vi "Hi_Tec_Control.vi"(2 "Carrier 1_50 Voltage":dbl(knob) min=0.0 max=5.0 scale=0.0..5.0 scale format="%.1f", 3 "Client Name":string, 4 "Trace_2 Voltage":dbl(knob) min=0.0 max=5.0 scale=0.0..5.0 scale format="%.1f", 5 "Trace Voltage":dbl(knob) min=0.0 max=5.0 scale=0.0..5.0 scale format="%.1f", 6 "Carrier 2 Voltage":dbl(knob) min=0.0 max=5.0 scale=0.0..5.0 scale format="%.1f", 7 "Carrier 1 Voltage":dbl(knob) min=0.0 max=5.0 scale=0.0..5.0 scale format="%.1f") -> (1 "Scan Comments":string)   [LabVIEW 2018]
uses:
  ADAM Client/Sub VIs/Channel_State_Control.ctl
  Anemometry/Anemometry Sub Vis/Controls/In_Range.ctl
  ADAM Client/Sub VIs/ADAM Controls/Update_scan_value.ctl
panel:
  out "Second stage":dbl[][](graph)
  out "First stage":dbl[][](graph)
  out "Increasing trace":bool
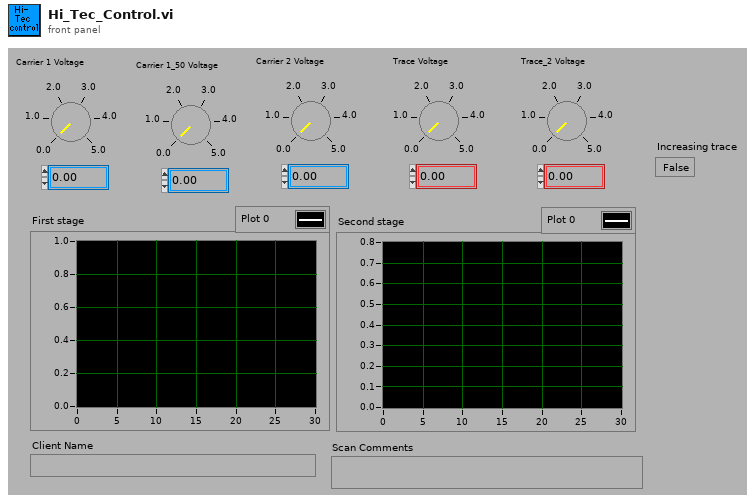
[diagram p1: front panel]
types:
  T1 = typedef "Channel_State_Control.ctl" = enum16{"Channel Name", "Channel Name Starts with", "Main Address"}
  T2 = typedef "In_Range.ctl" = enum16{"%", "±", "% & ±"}
  T3 = typedef "Update_scan_value.ctl" = cluster{"Channel Name":string, "New Value":dbl}
  T4 = enum16{"Append to Global", "Read Global then Clear"}
  T5 = typedef "Ch_description_ADAM.ctl" = cluster{"Ch Name":string, "Type":T6, "Function":T7, "Ch State":T8, "Calibration type":T9, "A":dbl, "B":dbl, "C":dbl, "D":dbl, "Comments":string, "Address":T10, "String":string, "Duty":u16}
  T6 = typedef "Module_type_ADAM.ctl" = string
  T7 = typedef "Function_ADAM.ctl" = enum16{"Analogue Input", "Digital Input", "Event counter", "Event rate", "Analogue Output", "Digital Output", "Relay Output"}
  T8 = typedef "Channel_State.ctl" = enum16{"On", "Off", "Always On", "Always Off"}
  T9 = typedef "Calib_type_ADAM.ctl" = string
  T10 = typedef "Address.ctl" = cluster{"Main":i32, "Ch.":i32, "Sub":i32, "Port Name":string}
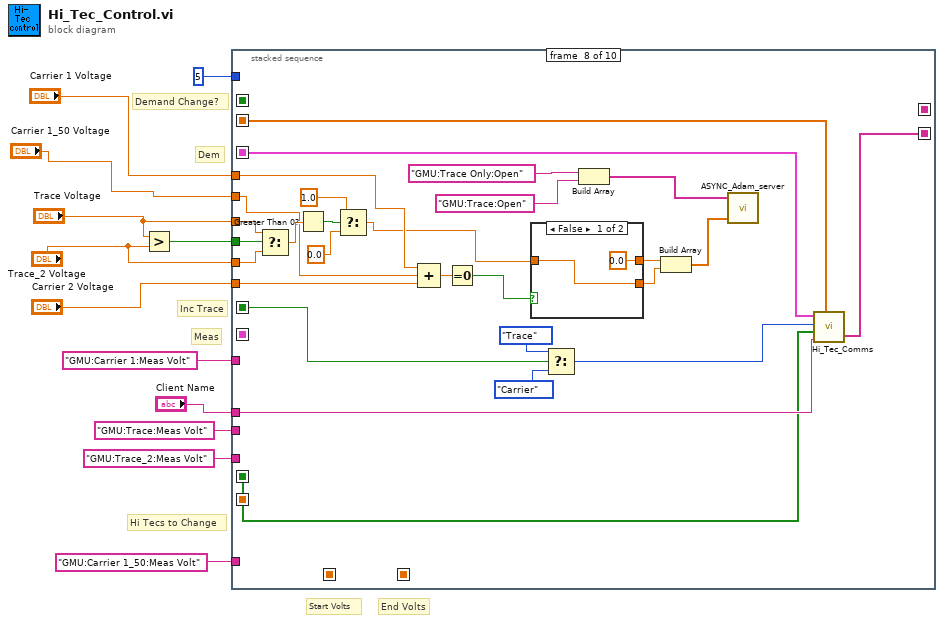
[diagram p0: block diagram]
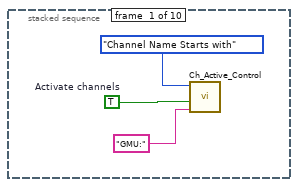
[diagram p2: hidden frame]
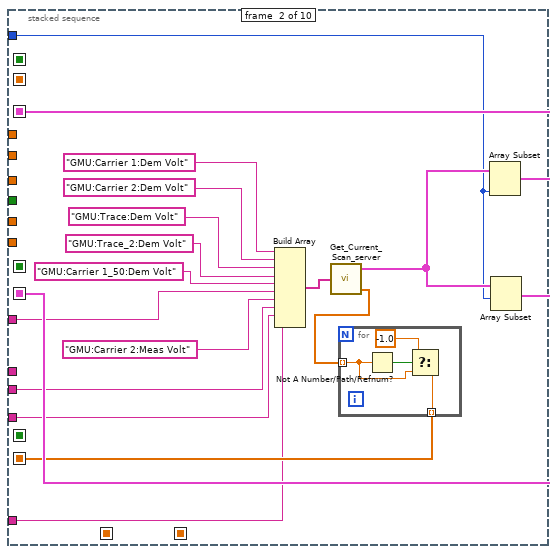
[diagram p3: hidden frame]
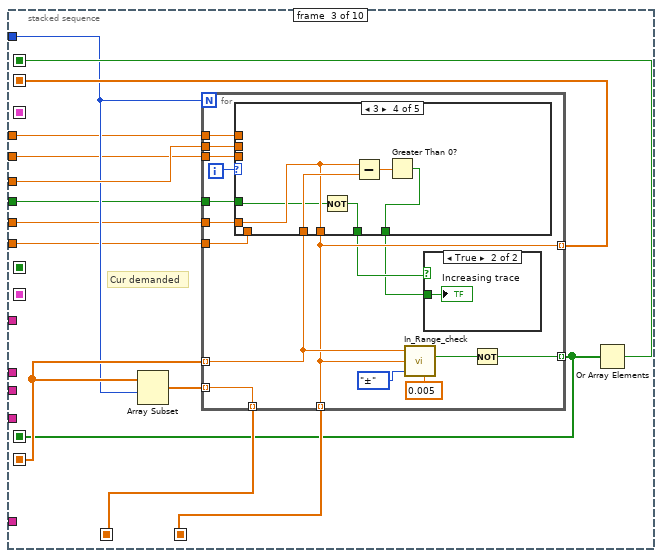
[diagram p4: hidden frame]
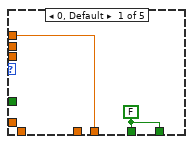
[diagram p6: hidden frame]
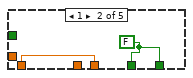
[diagram p7: hidden frame]
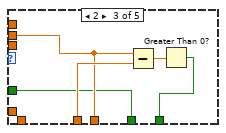
[diagram p8: hidden frame]
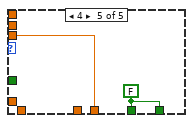
[diagram p9: hidden frame]
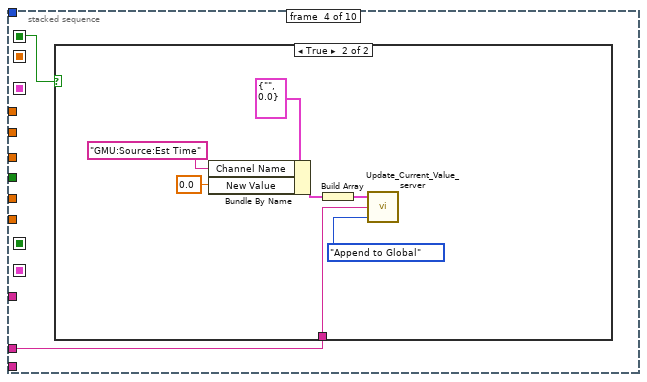
[diagram p10: hidden frame]
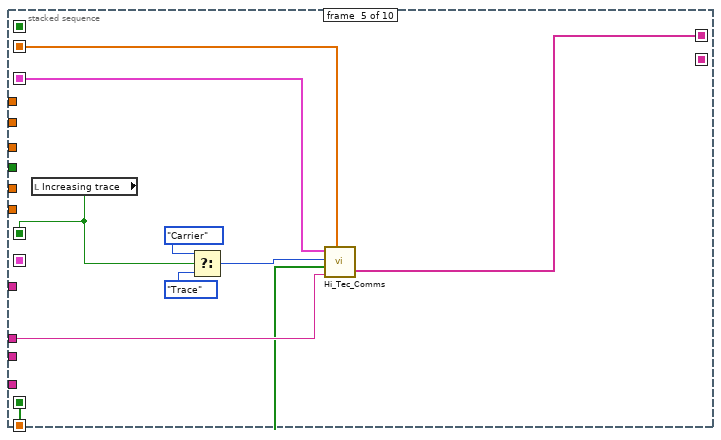
[diagram p12: hidden frame]
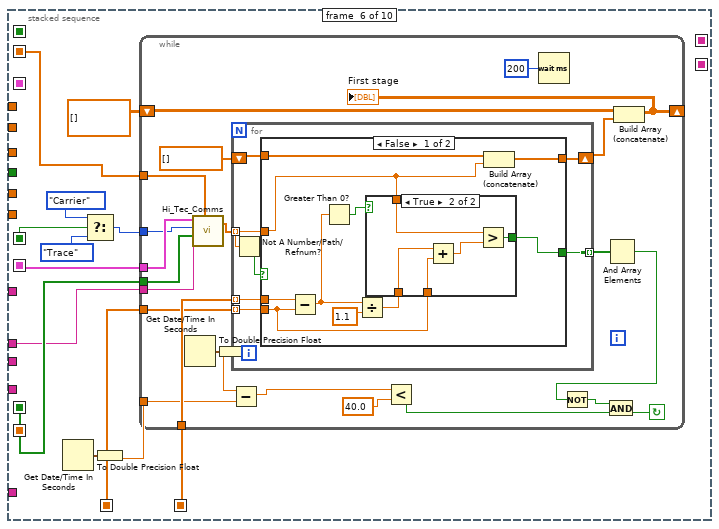
[diagram p13: hidden frame]
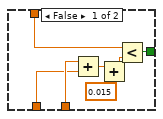
[diagram p14: hidden frame]
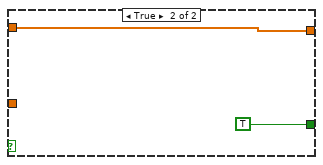
[diagram p15: hidden frame]
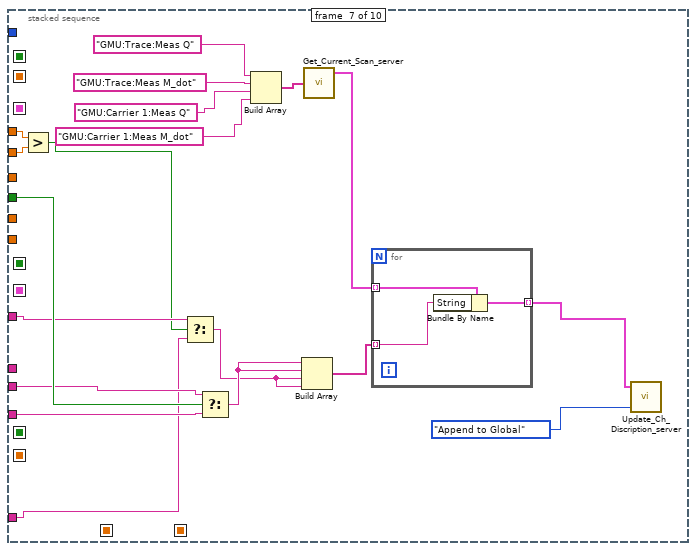
[diagram p16: hidden frame]
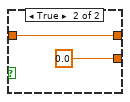
[diagram p17: hidden frame]
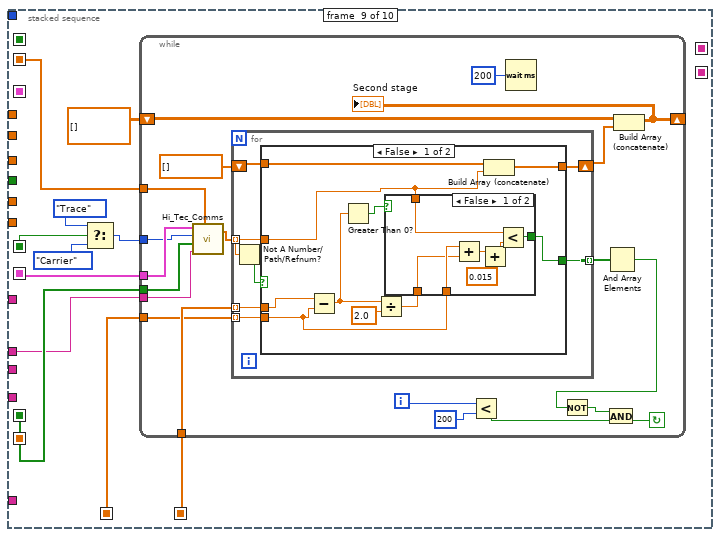
[diagram p18: hidden frame]
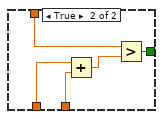
[diagram p19: hidden frame]
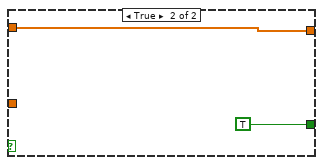
[diagram p20: hidden frame]
diagram:
  # "Dem"
  # "Demand Change?"
  # "End Volts"
  # "Start Volts"
  # "Inc Trace"
  # "Meas"
  # "Hi Tecs to Change"
  n1 = Greater?(x="Trace Voltage", y="Trace_2 Voltage") -> (0:w9:bool)
  n2 = stacked-sequence {
    seq-local: [_ w28 _ _ _ _ _ _ _ _] -> [_ _ _ _ w96 _ _ w208 _ w289]
    seq-local: [_ w23 _ _ _ _ _ _ _ _] -> [_ _ w48 _ _ _ _ _ _ _]
    seq-local: [_ _ w46 _ _ _ _ _ _ _] -> [_ _ _ _ w95 w115 _ w207 w234 _]
    seq-local: [_ w27 _ _ _ _ _ _ _ _] -> [_ _ _ _ _ w111 _ _ w230 _]
    seq-local: [_ _ _ _ w102 _ _ _ _ _] -> [_ _ _ _ _ w112 _ w219 w231 _]
    seq-local: [_ _ w50 _ _ _ _ _ _ _] -> [_ _ _ _ _ w108 _ _ w227 _]
    seq-local: [_ _ w49 _ _ _ _ _ _ _] -> [_ _ _ _ _ w109 _ _ w228 _]
    seq-local: [_ _ w45 _ _ _ _ _ _ _] -> [_ _ _ w85 _ _ _ _ _ _]
    seq-local: [_ _ w43 _ _ _ _ _ _ _] -> [_ _ _ _ w97 w103 _ w209 w224 w288]
    seq-local: [_ _ _ _ w94 _ _ _ _ _] -> [_ _ _ _ _ _ _ _ _ _]
    seq-local: [_ _ _ _ _ _ _ w206 _ _] -> [_ _ _ _ _ _ _ _ _ _]
    tunnel: "Client Name" -> [_ _ _ w86 w98 w105 _ w215 w225 w290]
    tunnel: "Trace Voltage" -> [_ _ w44 _ _ _ _ w204 _ _]
    tunnel: 5 ("Array Length") -> [_ w21 w42 _ _ _ _ _ _ _]
    tunnel: w9 -> [_ _ w41 _ _ _ w184 w205 _ _]
    tunnel: "Trace_2 Voltage" -> [_ _ w40 _ _ _ _ w202 _ _]
    tunnel: "GMU:Trace:Meas Volt" -> [_ w20 _ _ _ _ w183 _ _ _]
    tunnel: "GMU:Trace_2:Meas Volt" -> [_ w19 _ _ _ _ w182 _ _ _]
    tunnel: "Carrier 1 Voltage" -> [_ _ w39 _ _ _ w177 w199 _ _]
    tunnel: "Carrier 1_50 Voltage" -> [_ _ w38 _ _ _ w176 w200 _ _]
    tunnel: "GMU:Carrier 1:Meas Volt" -> [_ w17 _ _ _ _ w175 _ _ _]
    tunnel: "GMU:Carrier 1_50:Meas Volt" -> [_ w16 _ _ _ _ w174 _ _ _]
    tunnel: "Carrier 2 Voltage" -> [_ _ w37 _ _ _ _ w201 _ _]
    frame #0 {
      w13 = TRUE  # Activate channels
      n3 = call "Ch_Active_Control.vi"("Match"="GMU:", "Activate Channels?"=w13, "Control on"=Channel_State_Control."Channel Name Starts with") -> ()  [unwired: 1 in, 2 out]
    }
    frame #1 {
      n4 = Build Array("GMU:Carrier 1:Dem Volt", "GMU:Carrier 2:Dem Volt", "GMU:Trace:Dem Volt", "GMU:Trace_2:Dem Volt", "GMU:Carrier 1_50:Dem Volt", w17, "GMU:Carrier 2:Meas Volt", w20, w19, w16) -> (w32:string[])
      n5 = call "Get_Current_Scan_server.vi"("Desired Channels"=w32) -> ("Ch Description Array"=w26:T5[], "Numerical Values"=w24:dbl[])  [unwired: 1 out]
      n6 = for {
        tunnel: w24 -> [w35] mode=indexing
        tunnel: [w34] -> w23 mode=indexing
        n7 = Not A Number/Path/Refnum?(number/path/refnum=w35) -> (NaN/Path/Refnum?=w36:bool)
        n8 = Select(t=-1.0, s=w36, f=w35) -> (s? t:f=w34:dbl)
      }
      n9 = Array Subset(array=w26, length=w21) -> (w28:T5[])  [unwired: 1 in]
      n10 = Array Subset(array=w26, index=w21) -> (w27:T5[])  [unwired: 1 in]
    }
    frame #2 {
      # "Cur demanded"
      n11 = Array Subset(array=w48, index=w42) -> (w47:dbl[])  [unwired: 1 in]
      n12 = for {
        N: w42 -> [_]
        tunnel: w48 -> [w61] mode=indexing
        tunnel: [w64] -> w50 mode=indexing
        tunnel: [w58] -> w49 mode=indexing
        tunnel: [w65] -> w46 mode=indexing
        tunnel: w47 -> [w64] mode=indexing
        tunnel: w44 -> [w59]
        tunnel: [w58] -> w43 mode=indexing
        tunnel: w41 -> [w56]
        tunnel: w40 -> [w54]
        tunnel: w39 -> [w53]
        tunnel: w38 -> [w52]
        tunnel: w37 -> [w51]
        i -> [w66]
        n13 = case shown="3" w66 {
          tunnel: [w68 w70 w74 w79 w83] -> w58
          tunnel: w61 -> [_ _ w76 w82 _]
          tunnel: w59 -> [_ _ w74 _ _]
          tunnel: [w69 w71 w73 w77 w84] -> w57
          tunnel: w56 -> [_ _ w73 w78 _]
          tunnel: [w69 w71 w72 w80 w84] -> w55
          tunnel: w54 -> [_ _ _ w79 _]
          tunnel: w53 -> [w68 _ _ _ _]
          tunnel: w52 -> [_ _ _ _ w83]
          tunnel: w51 -> [_ w70 _ _ _]
          frame 0, Default {
            w69 = FALSE
          }
          frame 1 {
            w71 = FALSE
          }
          frame 2 {
            n14 = Subtract(x=w74, y=w76) -> (x-y=w75:dbl)
            n15 = Greater Than 0?(x=w75) -> (x > 0?=w72:bool)
          }
          frame 3 {
            n16 = Not(x=w78) -> (.not. x?=w77:bool)
            n17 = Subtract(x=w79, y=w82) -> (x-y=w81:dbl)
            n18 = Greater Than 0?(x=w81) -> (x > 0?=w80:bool)
          }
          frame 4 {
            w84 = FALSE
          }
        }
        n19 = call "In_Range_check.vi"("±"=0.005 ("%"), "Mode"=In_Range."±", "Value"=w58, "Setpoint"=w61) -> ("In Range"=w60:bool)  [unwired: 1 in, 2 out]
        n20 = case shown="True" w57 {
          tunnel: w55 -> [_ w67]
          frame False {
          }
          frame True {
            "Increasing trace" <- w67
          }
        }
        n21 = Not(x=w60) -> (.not. x?=w65:bool)
      }
      n22 = Or Array Elements(Boolean array=w46) -> (logical OR=w45:bool)
    }
    frame #3 {
      n23 = case shown="True" w85 {
        tunnel: w86 -> [_ w93]
        frame False {
        }
        frame True {
          n24 = Bundle By Name(cluster=T3 {"Channel Name"="", "New Value"=0.0} ("Update Scan Value Cluster"), "Channel Name"="GMU:Source:Est Time", "New Value"=0.0 ("Bundle Element")) -> (w88:T3)
          n25 = Build Array(w88) -> (w87:T3[])
          n26 = call "Update_Current_Value_server.vi"("Mode"=T4."Append to Global", "Client HD name"=w93, "Update array in"=w87) -> ()  [unwired: 1 out]
        }
      }
    }
    frame #4 {
      n27 = local read "Increasing trace"() -> (w102:bool)
      n28 = Select(t=enum16{"Carrier", "Trace"}."Carrier" ("Type"), s=w102, f=enum16{"Carrier", "Trace"}."Trace" ("Type")) -> (s? t:f=w99:enum16{"Carrier", "Trace"})
      n29 = call "Hi_Tec_Comms.vi"("Ch Description Array"=w96, "Type"=w99, "Hi Tec's To Change"=w95, "Client Name"=w98, "Dem Volts"=w97) -> ("Scan comments"=w94:string[])  [unwired: 1 out]
    }
    frame #5 {
      n30 = Get Date/Time In Seconds() -> (seconds since 1Jan1904=w104:timestamp)
      n31 = Select(t=enum16{"Carrier", "Trace"}."Carrier" ("Type"), s=w112, f=enum16{"Carrier", "Trace"}."Trace" ("Type")) -> (s? t:f=w110:enum16{"Carrier", "Trace"})
      n32 = To Double Precision Float(number=w104) -> (double precision float=w106:dbl)
      n33 = while {
        tunnel: w105 -> [w119]
        tunnel: w106 -> [w122]
        shift-left: dbl[][] [] -> [w128]
        shift-right: [w127] -> _
        tunnel: w108 -> [w135]
        tunnel: w109 -> [w136]
        tunnel: w110 -> [w137]
        tunnel: w111 -> [w138]
        tunnel: w115 -> [w129]
        tunnel: w103 -> [w116]
        stop <- w124 continue-if-true
        n34 = Get Date/Time In Seconds() -> (seconds since 1Jan1904=w118:timestamp)
        n35 = call "Hi_Tec_Comms.vi"("Ch Description Array"=w138, "Type"=w137, "Hi Tec's To Change"=w129, "Client Name"=w119, "Dem Volts"=w116) -> ("Outputs"=w134:dbl[])  [unwired: 1 out]
        n36 = To Double Precision Float(number=w118) -> (double precision float=w123:dbl)
        n37 = Subtract(x=w123, y=w122) -> (x-y=w121:dbl)
        n38 = for {
          tunnel: w136 -> [w145] mode=indexing
          tunnel: w135 -> [w144] mode=indexing
          tunnel: w134 -> [w140] mode=indexing
          tunnel: [w143] -> w133 mode=indexing
          shift-right: [w141] -> w130
          shift-left: dbl[] [] -> [w142]
          n39 = Not A Number/Path/Refnum?(number/path/refnum=w140) -> (NaN/Path/Refnum?=w139:bool)
          n40 = case shown="False" w139 {
            tunnel: w145 -> [w152 _]
            tunnel: w144 -> [w148 _]
            tunnel: w140 -> [w147 _]
            tunnel: [w146 TRUE] -> w143
            tunnel: w142 -> [w151 w168]
            tunnel: [w150 w168] -> w141
            frame False {
              n41 = Subtract(x=w152, y=w148) -> (x-y=w154:dbl)
              n42 = Greater Than 0?(x=w154) -> (x > 0?=w153:bool)
              n43 = Divide(x=w154, y=1.1) -> (x/y=w149:dbl)
              n44 = case shown="True" w153 {
                tunnel: w149 -> [w161 w167]
                tunnel: w148 -> [w162 w166]
                tunnel: w147 -> [w160 w164]
                tunnel: [w159 w163] -> w146
                frame False {
                  n45 = Add(x=w162, y=w161) -> (x+y=w158:dbl)
                  n46 = Add(x=w158, y=0.015 ("x")) -> (x+y=w157:dbl)
                  n47 = Less?(x=w160, y=w157) -> (x < y?=w159:bool)
                }
                frame True {
                  n48 = Add(x=w167, y=w166) -> (x+y=w165:dbl)
                  n49 = Greater?(x=w164, y=w165) -> (0:w163:bool)
                }
              }
              n50 = Build Array (concatenate)(w151, w147) -> (w150:dbl[])
            }
            frame True {
            }
          }
        }
        n51 = Less?(x=w121, y=40.0) -> (x < y?=w126:bool)
        n52 = Wait (ms)(milliseconds to wait=u32 200) -> ()  [unwired: 1 out]
        n53 = And Array Elements(Boolean array=w133) -> (logical AND=w132:bool)
        n54 = Not(x=w132) -> (.not. x?=w125:bool)
        n55 = And(x=w125, y=w126) -> (x .and. y?=w124:bool)
        n56 = Build Array (concatenate)(w128, w130) -> (w127:dbl[][])
        "First stage" <- w127
      }
    }
    frame #6 {
      n57 = Greater?(x=w177, y=w176) -> (0:w173:bool)
      n58 = Select(t=w175, s=w173, f=w174) -> (s? t:f=w172:string)
      n59 = Select(t=w183, s=w184, f=w182) -> (s? t:f=w178:string)
      n60 = Build Array("GMU:Trace:Meas Q", "GMU:Trace:Meas M_dot", "GMU:Carrier 1:Meas Q", "GMU:Carrier 1:Meas M_dot") -> (w186:string[])
      n61 = Build Array(w178, w178, w172, w172) -> (w171:string[])
      n62 = call "Get_Current_Scan_server.vi"("Desired Channels"=w186) -> ("Ch Description Array"=w185:T5[])  [unwired: 2 out]
      n63 = for {
        tunnel: w185 -> [w191] mode=indexing
        tunnel: w171 -> [w190] mode=indexing
        tunnel: [w189] -> w170 mode=indexing
        n64 = Bundle By Name(cluster=w191, "String"=w190) -> (w189:T5)
      }
      n65 = call "Update_Ch_Discription_server.vi"("Mode"=T4."Append to Global", "Channels to update In"=w170) -> ()  [unwired: 1 in, 1 out]
    }
    frame #7 {
      n66 = Select(t=w204, s=w205, f=w202) -> (s? t:f=w203:dbl)
      n67 = Greater Than 0?(x=w203) -> (x > 0?=w214:bool)
      n68 = Select(t=1.0, s=w214, f=0.0) -> (s? t:f=w194:dbl)
      n69 = Compound Arithmetic op=ADD(w199, w200, w201) -> (w198:dbl)
      n70 = Equal To 0?(x=w198) -> (x = 0?=w195:bool)
      n71 = case shown="False" w195 {
        tunnel: w194 -> [w221 w223]
        tunnel: [0.0 ("f") w223] -> w193
        tunnel: [w221 0.0 ("f")] -> w192
        frame False {
        }
        frame True {
        }
      }
      n72 = Select(t=enum16{"Carrier", "Trace"}."Trace" ("Type"), s=w219, f=enum16{"Carrier", "Trace"}."Carrier" ("Type")) -> (s? t:f=w216:enum16{"Carrier", "Trace"})
      n73 = Build Array("GMU:Trace Only:Open", "GMU:Trace:Open") -> (w211:string[])
      n74 = Build Array(w193, w192) -> (w210:dbl[])
      n75 = call "ASYNC_Adam_server.vi"("Values"=w210, "Channel Names"=w211) -> ()  [unwired: 2 in, 2 out]
      n76 = call "Hi_Tec_Comms.vi"("Ch Description Array"=w208, "Type"=w216, "Hi Tec's To Change"=w207, "Client Name"=w215, "Dem Volts"=w209) -> ("Scan comments"=w206:string[])  [unwired: 1 out]
    }
    frame #8 {
      n77 = Select(t=enum16{"Carrier", "Trace"}."Trace" ("Type"), s=w231, f=enum16{"Carrier", "Trace"}."Carrier" ("Type")) -> (s? t:f=w229:enum16{"Carrier", "Trace"})
      n78 = while {
        tunnel: w225 -> [w237]
        shift-left: dbl[][] [] -> [w244]
        shift-right: [w238] -> _
        tunnel: w227 -> [w251]
        tunnel: w228 -> [w252]
        tunnel: w229 -> [w253]
        tunnel: w230 -> [w254]
        tunnel: w234 -> [w245]
        tunnel: w224 -> [w235]
        i -> [w240]
        stop <- w239 continue-if-true
        n79 = call "Hi_Tec_Comms.vi"("Ch Description Array"=w254, "Type"=w253, "Hi Tec's To Change"=w245, "Client Name"=w237, "Dem Volts"=w235) -> ("Outputs"=w250:dbl[])  [unwired: 1 out]
        n80 = for {
          tunnel: w252 -> [w261] mode=indexing
          tunnel: w251 -> [w260] mode=indexing
          tunnel: w250 -> [w256] mode=indexing
          tunnel: [w259] -> w249 mode=indexing
          shift-right: [w257] -> w246
          shift-left: dbl[] [] -> [w258]
          n81 = Not A Number/Path/Refnum?(number/path/refnum=w256) -> (NaN/Path/Refnum?=w255:bool)
          n82 = case shown="False" w255 {
            tunnel: w261 -> [w265 _]
            tunnel: w260 -> [w264 _]
            tunnel: w256 -> [w263 _]
            tunnel: [w262 TRUE] -> w259
            tunnel: w258 -> [w271 w284]
            tunnel: [w270 w284] -> w257
            frame False {
              n83 = Subtract(x=w265, y=w264) -> (x-y=w268:dbl)
              n84 = Greater Than 0?(x=w268) -> (x > 0?=w267:bool)
              n85 = Divide(x=w268, y=2.0) -> (x/y=w266:dbl)
              n86 = case shown="False" w267 {
                tunnel: w266 -> [w277 w283]
                tunnel: w264 -> [w278 w282]
                tunnel: w263 -> [w276 w280]
                tunnel: [w275 w279] -> w262
                frame False {
                  n87 = Add(x=w278, y=w277) -> (x+y=w274:dbl)
                  n88 = Add(x=w274, y=0.015 ("x")) -> (x+y=w273:dbl)
                  n89 = Less?(x=w276, y=w273) -> (x < y?=w275:bool)
                }
                frame True {
                  n90 = Add(x=w283, y=w282) -> (x+y=w281:dbl)
                  n91 = Greater?(x=w280, y=w281) -> (0:w279:bool)
                }
              }
              n92 = Build Array (concatenate)(w271, w263) -> (w270:dbl[])
            }
            frame True {
            }
          }
        }
        n93 = Less?(x=w240, y=200) -> (x < y?=w242:bool)
        n94 = Wait (ms)(milliseconds to wait=u32 200) -> ()  [unwired: 1 out]
        n95 = And Array Elements(Boolean array=w249) -> (logical AND=w248:bool)
        n96 = Not(x=w248) -> (.not. x?=w241:bool)
        n97 = And(x=w241, y=w242) -> (x .and. y?=w239:bool)
        n98 = Build Array (concatenate)(w244, w246) -> (w238:dbl[][])
        "Second stage" <- w238
      }
    }
    frame #9 {
      # "Make Sure all the Hi-Tec demands have been set, even increments of less than 0.045 volts"
      n99 = for {
        tunnel: w289 -> [w295] mode=indexing
        tunnel: w290 -> [w293]
        tunnel: w288 -> [w294] mode=indexing
        tunnel: [w292] -> w287 mode=indexing
        n100 = for {
          N: 10 -> [_]
          tunnel: w295 -> [w300]
          tunnel: w294 -> [w299]
          tunnel: w293 -> [w298]
          tunnel: [w297] -> w292
          stop <- w296 stop-if-true
          n101 = call "Adam_Ch_Input_Output_ASYNC.vi"("Client Name"=w298, "Value to Output"=w299, "Ch Description"=w300) -> ("Scan comment"=w297:string)  [unwired: 4 in, 4 out]
          n102 = Empty String/Path?(string/path=w297) -> (empty?=w296:bool)
          n103 = case shown="False" w296 {
            frame False {
              n104 = Wait (ms)(milliseconds to wait=u32 500) -> ()  [unwired: 1 out]
            }
            frame True {
            }
          }
        }
      }
      n105 = Concatenate Strings(w287) -> (→"Scan Comments":string)
    }
  }
